vi "slice_expt_to_XYs.vi"(8 "error in (no error)":errorcluster, 9 "Y channel":i32=7, 10 "X channel":i32=12, 11 "All expt data":dbl[][][](array[numeric])) -> (0 "error out":errorcluster, 3 "Array":T1(array[cluster]))   [LabVIEW 2016]
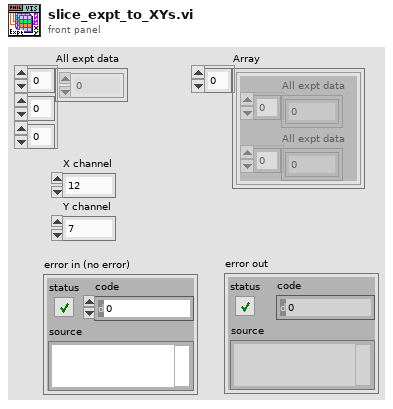
[diagram p1: front panel]
types:
  T1 = cluster{"All expt data":dbl[], "All expt data":dbl[]}[]
  T2 = cluster{"All expt data":dbl[], "All expt data":dbl[]}
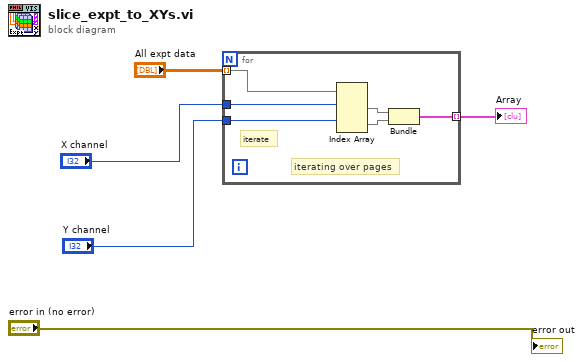
[diagram p0: block diagram]
diagram:
  n1 = for {
    tunnel: "All expt data" -> [w11] mode=indexing
    tunnel: [w9] -> w4 mode=indexing
    tunnel: "X channel" -> [w7]
    tunnel: "Y channel" -> [w6]
    # "iterating over pages"
    # "iterate"
    n2 = Index Array(array=w11, index (row) #1=w7, index (row) #2=w6) -> (element #1=w8:dbl[], element #2=w10:dbl[])  [unwired: 2 in]
    n3 = Bundle("All expt data"=w8, "All expt data"=w10) -> (w9:T2)  [unwired: 1 in]
  }
  "Array" <- w4
  "error out" <- "error in (no error)"
